vi "glueAlignPinInsert.vi"() -> ()   [LabVIEW 2015]
uses:
  GlobalPath.vi
  GlobalData.vi
  GlobalVi.vi
panel:
  in  "ptfe 41":bool caption="Manually push down the two pins of the vertical positioning tool to insert them in the holes of the plates"
  out "PanelName":string
  in  "ptfe 33":bool caption="Remove the electroerosion pin and the precision rod"
  in  "ptfe 10":bool caption="Place and screw the blocking plate to the vertical positioning tool to keep the pin orthogonality during the curing of the glue"
  in  "ptfe 40":bool caption="Insert the electroerosition pin in the slotted insert and the precision rod in the circular insert"
  in  "ptfe 38":bool caption="Check the planarity of the tool with the gauge machine"
  in  "ptfe 37":bool caption="Tighten the three screws to block the vertical positioning tool in place"
  in  "ptfe 35":bool caption="Position the vertical positioning tool on the reference plate against with its positioning pins"
  in  "ptfe 34":bool caption="Deposit the glue on the stainless steel slotted and circular insert groove"
  in  "ptfe 32":bool caption="Position the two inserts in the dedicated holes on the panel"
  in  "ptfe 26":bool caption="Position the panel on the table"
  in  "ptfe 25":bool caption="Move the panel away from the table"
  in  "ptfe 24":bool caption="Lift the panel from the table"
  in  "ptfe 23":bool caption="Switch on the vacuum on the machine"
  in  "ptfe 22":bool caption="Lower the machine on the panel"
  in  "ptfe 21":bool caption="Move the rotating machine on top of the panel"
  in  "Done ?":bool
  in  "ptfe 20":bool caption="Wait 24h for the glue to cure"
  in  "ptfe 19":bool caption="Position the reinforcing washers on the emerging part of the alignment inserts"
  in  "ptfe 18":bool caption="Deposit the glue on the emerging part of the alignment inserts using a thin needle"
  in  "ptfe 17":bool caption="Rotate the panel so that it's back side is up"
  in  "ptfe 16":bool caption="Switch off the vacuum"
  in  "ptfe 15":bool caption="Remove the three vertical positioning tools, blocking plates and positioning pins"
  in  "ptfe 14":bool caption="Wait 24h for the glue to cure"
  in  "ptfe 2":bool caption="Check that the vacuum is on"
  # "Gluing of Alignment Pin/Insert"
  # "ETA PANEL \nINSTRUCTIONS"
  # "GLUING OF THE SLOTTED BRASS AND CIRCULAR BRASS INSERT"
  # "Add info on enumeration"
  # "COMMON PROCEDURE"
  # "GLUE CURING OF THE TWO PINS AND INSERT"
  # "GLUING OF REINFORCING WASHERS ON PANEL BACK SIDE"
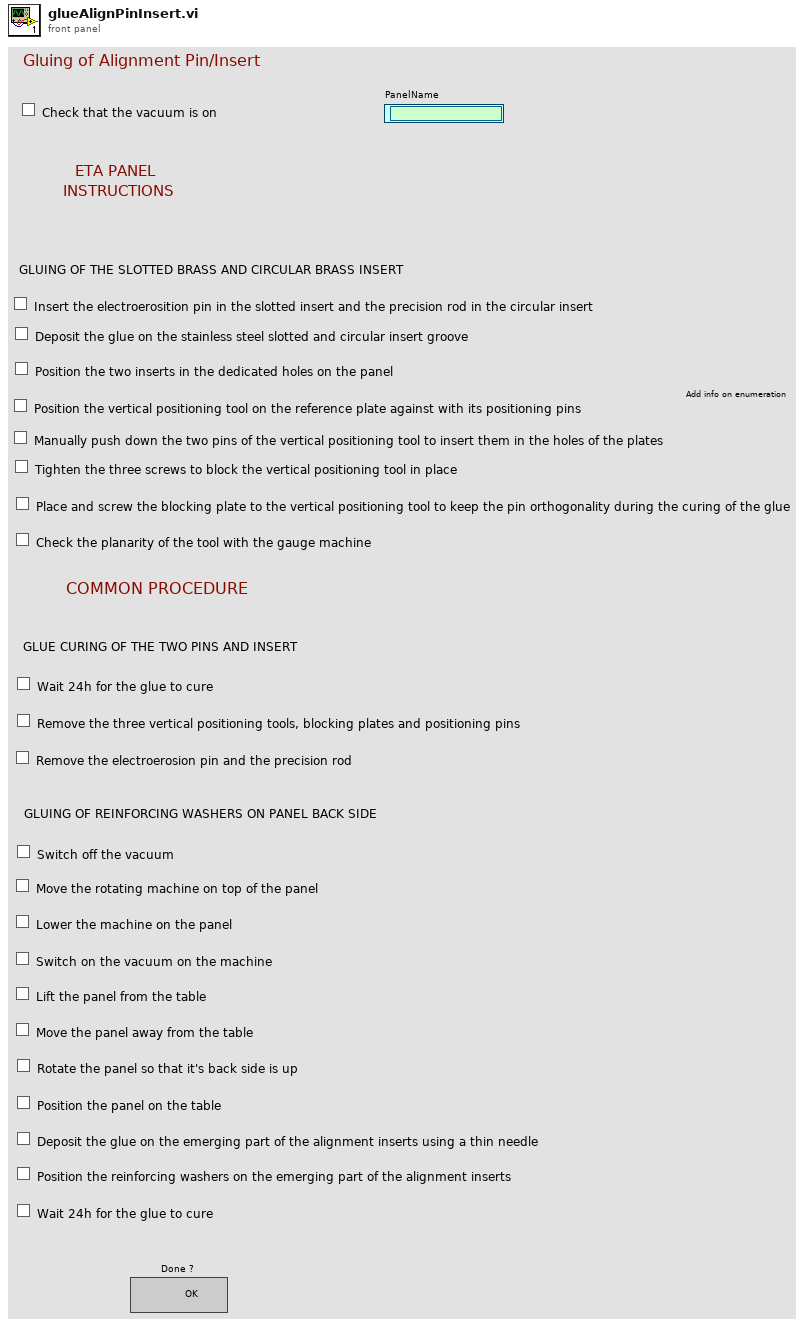
[diagram p1: front panel]
types:
  T1 = enum16{"open", "replace", "create", "open or create", "replace or create", "replace or create with confirmation"}
  T2 = enum32{"Bad", "Idle", "Run top level", "Running"}
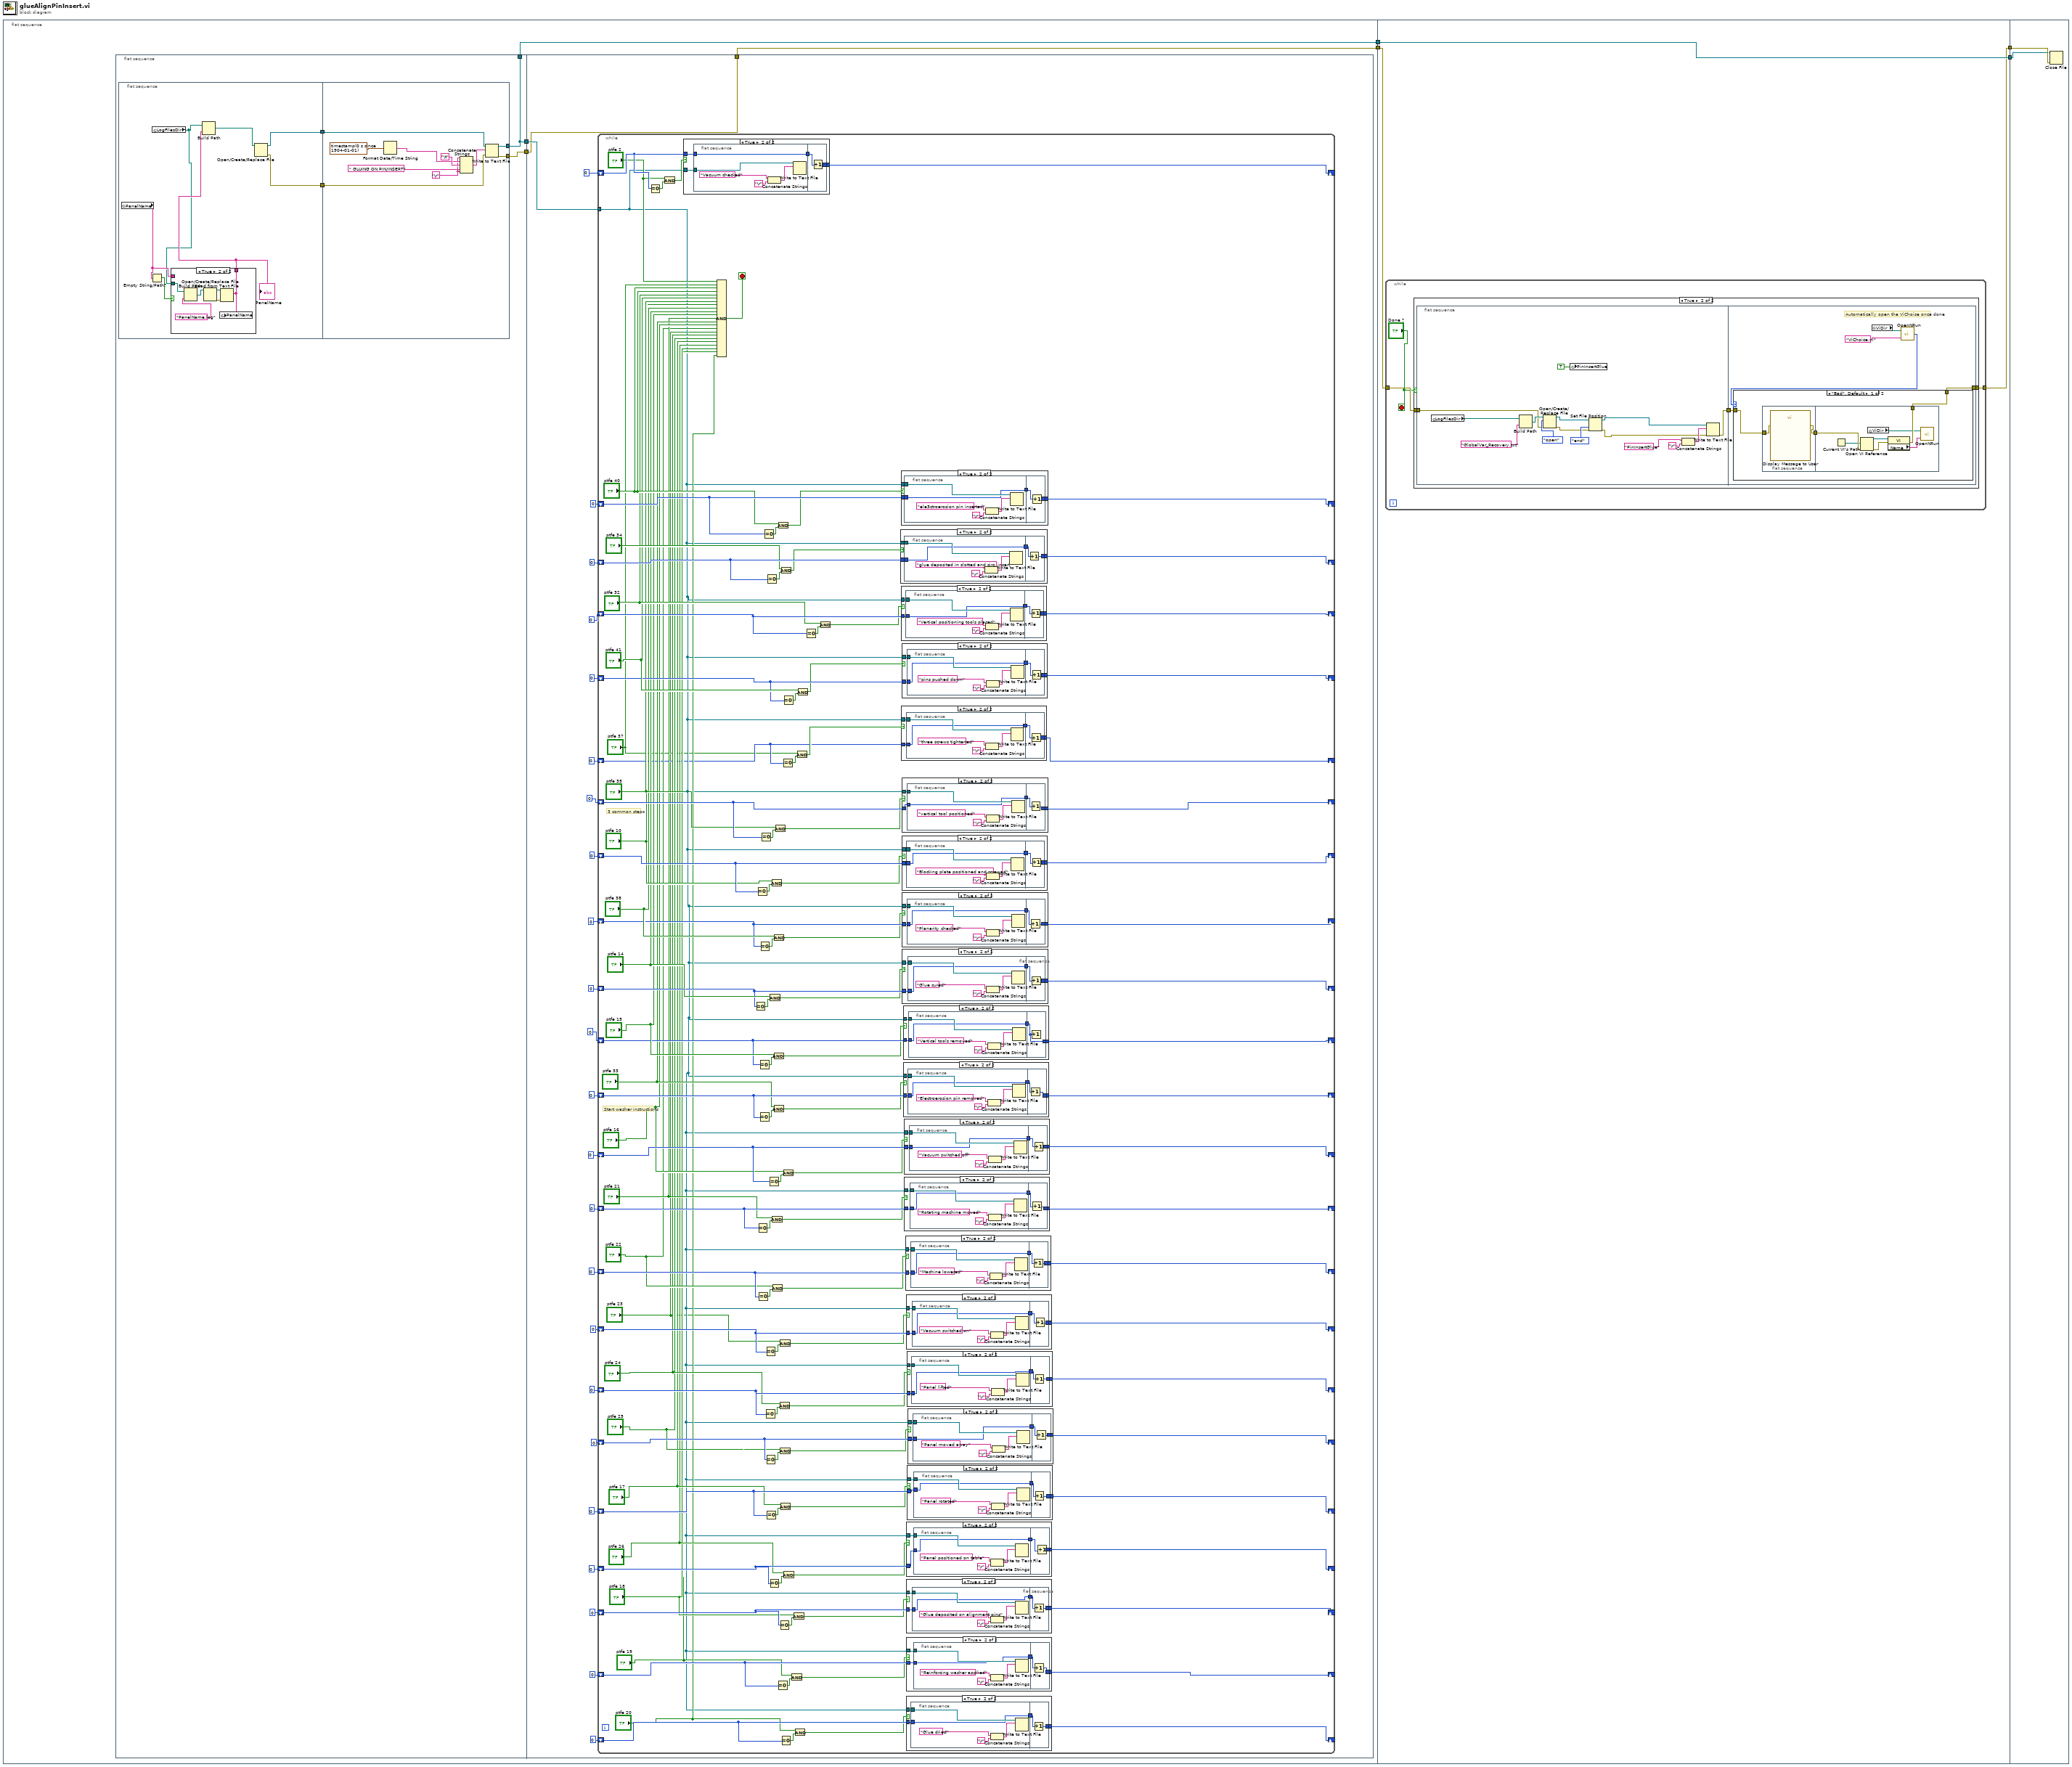
[diagram p0: block diagram]
diagram:
  n1 = flat-sequence {
    tunnel: [w5] -> w3
    tunnel: [w7] -> w2
    tunnel: [w454] -> w4
    tunnel: w3 -> [w455]
    tunnel: w2 -> [w456]
    tunnel: [w456] -> w1
    tunnel: w4 -> [w500]
    tunnel: w1 -> [w499]
    frame #0 {
      n2 = flat-sequence {
        tunnel: [w11] -> w8
        tunnel: [w11] -> w7
        tunnel: [w9] -> w6
        tunnel: w8 -> [w61]
        tunnel: w6 -> [w60]
        tunnel: [w60] -> w5
        frame #0 {
          n3 = flat-sequence {
            tunnel: [w18] -> w12
            tunnel: [w17] -> w10
            tunnel: w12 -> [w31]
            tunnel: [w30] -> w11
            tunnel: [w29] -> w9
            tunnel: w10 -> [w28]
            frame #0 {
              n4 = global read "GlobalData.vi" "PanelName"() -> (w16:string)
              n5 = Empty String/Path?(string/path=w16) -> (empty?=w15:bool)
              n6 = global read "GlobalPath.vi" "LogFilesDir"() -> (w13:path)
              n7 = case shown="True" w15 {
                tunnel: w13 -> [_ w26]
                tunnel: [w20 w21] -> w14
                tunnel: w16 -> [w20 _]
                frame False {
                }
                frame True {
                  n8 = Build Path(base path=w26, name or relative path="PanelName.log") -> (appended path=w25:path)
                  n9 = Open/Create/Replace File(file path (use dialog)=w25) -> (refnum out=w22:refnum<file>, error out=w23:errorcluster)  [unwired: 5 in, 1 out]
                  n10 = Read from Text File(file (use dialog)=w22, error in=w23) -> (text=w21:string)  [unwired: 2 in, 3 out]
                  n11 = global write "GlobalData.vi" "PanelName"(w21) -> ()
                }
              }
              "PanelName" <- w14
              n12 = Build Path(base path=w13, name or relative path=w14) -> (appended path=w19:path)
              n13 = Open/Create/Replace File(file path (use dialog)=w19) -> (refnum out=w18:refnum<file>, error out=w17:errorcluster)  [unwired: 5 in, 1 out]
            }
            frame #1 {
              w27 = "\r"
              n14 = Format Date/Time String(seconds (now)=timestamp(0 s since 1904-01-01)) -> (date/time string=w34:string)  [unwired: 2 in]
              n15 = Concatenate Strings(w27, w34, "\t", " GLUING ON PIN/INSERT", w27) -> (w32:string)
              n16 = Write to Text File(file (use dialog)=w31, text=w32, error in=w28) -> (refnum out=w30:refnum<file>, error out=w29:errorcluster)  [unwired: 1 in, 1 out]
            }
          }
        }
        frame #1 {
          n17 = while {
            tunnel: w61 -> [w67]
            shift-right: [w177] -> _
            shift-left: 0 -> [w154]
            shift-right: [w176] -> _
            shift-left: 0 -> [w146]
            shift-right: [w175] -> _
            shift-left: 0 -> [w145]
            shift-right: [w174] -> _
            shift-left: 0 -> [w144]
            shift-right: [w173] -> _
            shift-left: 0 -> [w136]
            shift-right: [w172] -> _
            shift-left: 0 -> [w134]
            shift-right: [w171] -> _
            shift-left: 0 -> [w126]
            shift-right: [w170] -> _
            shift-left: 0 -> [w122]
            shift-right: [w169] -> _
            shift-left: 0 -> [w119]
            shift-right: [w168] -> _
            shift-left: 0 -> [w116]
            shift-right: [w167] -> _
            shift-left: 0 -> [w114]
            shift-right: [w166] -> _
            shift-left: 0 -> [w103]
            shift-right: [w165] -> _
            shift-left: 0 -> [w102]
            shift-right: [w164] -> _
            shift-left: 0 -> [w101]
            shift-right: [w163] -> _
            shift-left: 0 -> [w100]
            shift-right: [w162] -> _
            shift-left: 0 -> [w99]
            shift-right: [w161] -> _
            shift-left: 0 -> [w98]
            shift-right: [w160] -> _
            shift-left: 0 -> [w97]
            shift-right: [w159] -> _
            shift-left: 0 -> [w96]
            shift-right: [w158] -> _
            shift-left: 0 -> [w95]
            shift-right: [w157] -> _
            shift-left: 0 -> [w75]
            shift-right: [w156] -> _
            shift-left: 0 -> [w74]
            shift-right: [w65] -> _
            shift-left: 0 -> [w66]
            stop <- w178 stop-if-true
            # "3 common steps"
            # "Start washer instructions"
            n18 = Equal To 0?(x=w154) -> (x = 0?=w155:bool)
            n19 = And(x="ptfe 2", y=w155) -> (x .and. y?=w152:bool)
            n20 = case shown="True" w152 {
              tunnel: w67 -> [_ w446]
              tunnel: w154 -> [w442 w445]
              tunnel: [w442 w443] -> w177
              frame False {
              }
              frame True {
                n21 = flat-sequence {
                  tunnel: w446 -> [w448]
                  tunnel: w445 -> [w447]
                  tunnel: [w447] -> w444
                  tunnel: w444 -> [w453]
                  tunnel: [w452] -> w443
                  frame #0 {
                    n22 = Concatenate Strings("Vacuum checked", "\r") -> (w451:string)
                    n23 = Write to Text File(file (use dialog)=w448, text=w451) -> ()  [unwired: 2 in, 3 out]
                  }
                  frame #1 {
                    n24 = Increment(x=w453) -> (x+1=w452:i32)
                  }
                }
              }
            }
            n25 = Compound Arithmetic op=AND("ptfe 2", "ptfe 37", "ptfe 40", "ptfe 40", "ptfe 32", "ptfe 41", "ptfe 35", "ptfe 10", "ptfe 38", "ptfe 14", "ptfe 15", "ptfe 21", "ptfe 33", "ptfe 16", "ptfe 22", "ptfe 23", "ptfe 24", "ptfe 25", "ptfe 17", "ptfe 26", "ptfe 18", "ptfe 19", "ptfe 20") -> (w178:bool)
            n26 = Equal To 0?(x=w119) -> (x = 0?=w129:bool)
            n27 = Equal To 0?(x=w126) -> (x = 0?=w131:bool)
            n28 = Equal To 0?(x=w102) -> (x = 0?=w111:bool)
            n29 = Equal To 0?(x=w101) -> (x = 0?=w110:bool)
            n30 = Equal To 0?(x=w116) -> (x = 0?=w128:bool)
            n31 = Equal To 0?(x=w114) -> (x = 0?=w127:bool)
            n32 = Equal To 0?(x=w122) -> (x = 0?=w130:bool)
            n33 = Equal To 0?(x=w134) -> (x = 0?=w147:bool)
            n34 = Equal To 0?(x=w146) -> (x = 0?=w151:bool)
            n35 = Equal To 0?(x=w99) -> (x = 0?=w108:bool)
            n36 = Equal To 0?(x=w100) -> (x = 0?=w109:bool)
            n37 = Equal To 0?(x=w98) -> (x = 0?=w107:bool)
            n38 = Equal To 0?(x=w97) -> (x = 0?=w106:bool)
            n39 = Equal To 0?(x=w145) -> (x = 0?=w150:bool)
            n40 = Equal To 0?(x=w103) -> (x = 0?=w112:bool)
            n41 = Equal To 0?(x=w96) -> (x = 0?=w105:bool)
            n42 = And(x="ptfe 14", y=w129) -> (x .and. y?=w118:bool)
            n43 = And(x="ptfe 10", y=w131) -> (x .and. y?=w124:bool)
            n44 = And(x="ptfe 21", y=w111) -> (x .and. y?=w90:bool)
            n45 = And(x="ptfe 22", y=w110) -> (x .and. y?=w88:bool)
            n46 = And(x="ptfe 15", y=w128) -> (x .and. y?=w115:bool)
            n47 = And(x="ptfe 33", y=w127) -> (x .and. y?=w113:bool)
            n48 = And(x="ptfe 38", y=w130) -> (x .and. y?=w121:bool)
            n49 = And(x="ptfe 35", y=w147) -> (x .and. y?=w132:bool)
            n50 = Equal To 0?(x=w75) -> (x = 0?=w77:bool)
            n51 = And(x="ptfe 40", y=w151) -> (x .and. y?=w142:bool)
            n52 = And(x="ptfe 24", y=w108) -> (x .and. y?=w86:bool)
            n53 = Equal To 0?(x=w95) -> (x = 0?=w104:bool)
            n54 = And(x="ptfe 23", y=w109) -> (x .and. y?=w62:bool)
            n55 = And(x="ptfe 25", y=w107) -> (x .and. y?=w84:bool)
            n56 = And(x="ptfe 17", y=w106) -> (x .and. y?=w82:bool)
            n57 = Equal To 0?(x=w74) -> (x = 0?=w76:bool)
            n58 = And(x="ptfe 34", y=w150) -> (x .and. y?=w140:bool)
            n59 = Equal To 0?(x=w66) -> (x = 0?=w69:bool)
            n60 = Equal To 0?(x=w136) -> (x = 0?=w148:bool)
            n61 = And(x="ptfe 16", y=w112) -> (x .and. y?=w92:bool)
            n62 = And(x="ptfe 26", y=w105) -> (x .and. y?=w80:bool)
            n63 = And(x="ptfe 19", y=w77) -> (x .and. y?=w73:bool)
            n64 = And(x="ptfe 18", y=w104) -> (x .and. y?=w78:bool)
            n65 = And(x="ptfe 20", y=w76) -> (x .and. y?=w72:bool)
            n66 = And(x="ptfe 37", y=w69) -> (x .and. y?=w68:bool)
            n67 = And(x="ptfe 41", y=w148) -> (x .and. y?=w135:bool)
            n68 = Equal To 0?(x=w144) -> (x = 0?=w149:bool)
            n69 = And(x="ptfe 32", y=w149) -> (x .and. y?=w139:bool)
            n70 = case shown="True" w140 {
              tunnel: w67 -> [_ w422]
              tunnel: w145 -> [w418 w420]
              tunnel: [w418 w419] -> w175
              frame False {
              }
              frame True {
                n71 = flat-sequence {
                  tunnel: w422 -> [w424]
                  tunnel: [w423] -> w421
                  tunnel: w420 -> [w423]
                  tunnel: w421 -> [w429]
                  tunnel: [w428] -> w419
                  frame #0 {
                    n72 = Concatenate Strings("glue deposited in slotted and circ. insert", "\r") -> (w427:string)
                    n73 = Write to Text File(file (use dialog)=w424, text=w427) -> ()  [unwired: 2 in, 3 out]
                  }
                  frame #1 {
                    n74 = Increment(x=w429) -> (x+1=w428:i32)
                  }
                }
              }
            }
            n75 = case shown="True" w142 {
              tunnel: w67 -> [_ w434]
              tunnel: w146 -> [w430 w433]
              tunnel: [w430 w431] -> w176
              frame False {
              }
              frame True {
                n76 = flat-sequence {
                  tunnel: w434 -> [w436]
                  tunnel: w433 -> [w435]
                  tunnel: [w435] -> w432
                  tunnel: w432 -> [w441]
                  tunnel: [w440] -> w431
                  frame #0 {
                    n77 = Concatenate Strings("ele3ctroerosion pin inserted", "\r") -> (w439:string)
                    n78 = Write to Text File(file (use dialog)=w436, text=w439) -> ()  [unwired: 2 in, 3 out]
                  }
                  frame #1 {
                    n79 = Increment(x=w441) -> (x+1=w440:i32)
                  }
                }
              }
            }
            n80 = case shown="True" w139 {
              tunnel: w67 -> [_ w410]
              tunnel: w144 -> [w406 w408]
              tunnel: [w406 w407] -> w174
              frame False {
              }
              frame True {
                n81 = flat-sequence {
                  tunnel: w410 -> [w412]
                  tunnel: [w411] -> w409
                  tunnel: w408 -> [w411]
                  tunnel: w409 -> [w417]
                  tunnel: [w416] -> w407
                  frame #0 {
                    n82 = Concatenate Strings("Vertical positioning tools placed", "\r") -> (w415:string)
                    n83 = Write to Text File(file (use dialog)=w412, text=w415) -> ()  [unwired: 2 in, 3 out]
                  }
                  frame #1 {
                    n84 = Increment(x=w417) -> (x+1=w416:i32)
                  }
                }
              }
            }
            n85 = case shown="True" w68 {
              tunnel: w67 -> [_ w183]
              tunnel: w66 -> [w179 w181]
              tunnel: [w179 w180] -> w65
              frame False {
              }
              frame True {
                n86 = flat-sequence {
                  tunnel: w183 -> [w185]
                  tunnel: [w184] -> w182
                  tunnel: w181 -> [w184]
                  tunnel: w182 -> [w190]
                  tunnel: [w189] -> w180
                  frame #0 {
                    n87 = Concatenate Strings("three screws tightened", "\r") -> (w188:string)
                    n88 = Write to Text File(file (use dialog)=w185, text=w188) -> ()  [unwired: 2 in, 3 out]
                  }
                  frame #1 {
                    n89 = Increment(x=w190) -> (x+1=w189:i32)
                  }
                }
              }
            }
            n90 = case shown="True" w135 {
              tunnel: w67 -> [_ w362]
              tunnel: w136 -> [w358 w360]
              tunnel: [w358 w359] -> w173
              frame False {
              }
              frame True {
                n91 = flat-sequence {
                  tunnel: w362 -> [w364]
                  tunnel: [w363] -> w361
                  tunnel: w360 -> [w363]
                  tunnel: w361 -> [w369]
                  tunnel: [w368] -> w359
                  frame #0 {
                    n92 = Concatenate Strings("pins pushed down", "\r") -> (w367:string)
                    n93 = Write to Text File(file (use dialog)=w364, text=w367) -> ()  [unwired: 2 in, 3 out]
                  }
                  frame #1 {
                    n94 = Increment(x=w369) -> (x+1=w368:i32)
                  }
                }
              }
            }
            n95 = case shown="True" w124 {
              tunnel: w67 -> [_ w386]
              tunnel: w126 -> [w382 w385]
              tunnel: [w382 w383] -> w171
              frame False {
              }
              frame True {
                n96 = flat-sequence {
                  tunnel: w386 -> [w388]
                  tunnel: w385 -> [w387]
                  tunnel: [w387] -> w384
                  tunnel: w384 -> [w393]
                  tunnel: [w392] -> w383
                  frame #0 {
                    n97 = Concatenate Strings("Blocking plate positioned and screwed", "\r") -> (w391:string)
                    n98 = Write to Text File(file (use dialog)=w388, text=w391) -> ()  [unwired: 2 in, 3 out]
                  }
                  frame #1 {
                    n99 = Increment(x=w393) -> (x+1=w392:i32)
                  }
                }
              }
            }
            n100 = case shown="True" w132 {
              tunnel: w67 -> [_ w398]
              tunnel: w134 -> [w394 w397]
              tunnel: [w394 w395] -> w172
              frame False {
              }
              frame True {
                n101 = flat-sequence {
                  tunnel: w398 -> [w400]
                  tunnel: w397 -> [w399]
                  tunnel: [w399] -> w396
                  tunnel: w396 -> [w405]
                  tunnel: [w404] -> w395
                  frame #0 {
                    n102 = Concatenate Strings("vertical tool positioned", "\r") -> (w403:string)
                    n103 = Write to Text File(file (use dialog)=w400, text=w403) -> ()  [unwired: 2 in, 3 out]
                  }
                  frame #1 {
                    n104 = Increment(x=w405) -> (x+1=w404:i32)
                  }
                }
              }
            }
            n105 = case shown="True" w121 {
              tunnel: w67 -> [_ w374]
              tunnel: w122 -> [w370 w372]
              tunnel: [w370 w371] -> w170
              frame False {
              }
              frame True {
                n106 = flat-sequence {
                  tunnel: w374 -> [w376]
                  tunnel: [w375] -> w373
                  tunnel: w372 -> [w375]
                  tunnel: w373 -> [w381]
                  tunnel: [w380] -> w371
                  frame #0 {
                    n107 = Concatenate Strings("Planarity checked", "\r") -> (w379:string)
                    n108 = Write to Text File(file (use dialog)=w376, text=w379) -> ()  [unwired: 2 in, 3 out]
                  }
                  frame #1 {
                    n109 = Increment(x=w381) -> (x+1=w380:i32)
                  }
                }
              }
            }
            n110 = case shown="True" w118 {
              tunnel: w67 -> [_ w350]
              tunnel: w119 -> [w346 w348]
              tunnel: [w346 w347] -> w169
              frame False {
              }
              frame True {
                n111 = flat-sequence {
                  tunnel: w350 -> [w352]
                  tunnel: [w351] -> w349
                  tunnel: w348 -> [w351]
                  tunnel: w349 -> [w357]
                  tunnel: [w356] -> w347
                  frame #0 {
                    n112 = Concatenate Strings("Glue cured", "\r") -> (w355:string)
                    n113 = Write to Text File(file (use dialog)=w352, text=w355) -> ()  [unwired: 2 in, 3 out]
                  }
                  frame #1 {
                    n114 = Increment(x=w357) -> (x+1=w356:i32)
                  }
                }
              }
            }
            n115 = case shown="True" w115 {
              tunnel: w67 -> [_ w339]
              tunnel: w116 -> [w335 w337]
              tunnel: [w335 w336] -> w168
              frame False {
              }
              frame True {
                n116 = flat-sequence {
                  tunnel: w339 -> [w341]
                  tunnel: [w340] -> w338
                  tunnel: w337 -> [w340]
                  tunnel: w338 -> [w345]
                  tunnel: [w345] -> w336
                  frame #0 {
                    n117 = Concatenate Strings("Vertical tools removed", "\r") -> (w344:string)
                    n118 = Write to Text File(file (use dialog)=w341, text=w344) -> ()  [unwired: 2 in, 3 out]
                  }
                  frame #1 {
                    n119 = Increment(x=w345) -> ()  [unwired: 1 out]
                  }
                }
              }
            }
            n120 = case shown="True" w113 {
              tunnel: w67 -> [_ w327]
              tunnel: w114 -> [w323 w325]
              tunnel: [w323 w324] -> w167
              frame False {
              }
              frame True {
                n121 = flat-sequence {
                  tunnel: w327 -> [w329]
                  tunnel: [w328] -> w326
                  tunnel: w325 -> [w328]
                  tunnel: w326 -> [w334]
                  tunnel: [w333] -> w324
                  frame #0 {
                    n122 = Concatenate Strings("Electroerosion pin removed", "\r") -> (w332:string)
                    n123 = Write to Text File(file (use dialog)=w329, text=w332) -> ()  [unwired: 2 in, 3 out]
                  }
                  frame #1 {
                    n124 = Increment(x=w334) -> (x+1=w333:i32)
                  }
                }
              }
            }
            n125 = case shown="True" w92 {
              tunnel: w67 -> [_ w315]
              tunnel: w103 -> [w311 w313]
              tunnel: [w311 w312] -> w166
              frame False {
              }
              frame True {
                n126 = flat-sequence {
                  tunnel: w315 -> [w317]
                  tunnel: [w316] -> w314
                  tunnel: w313 -> [w316]
                  tunnel: w314 -> [w322]
                  tunnel: [w321] -> w312
                  frame #0 {
                    n127 = Concatenate Strings("Vacuum switched off", "\r") -> (w320:string)
                    n128 = Write to Text File(file (use dialog)=w317, text=w320) -> ()  [unwired: 2 in, 3 out]
                  }
                  frame #1 {
                    n129 = Increment(x=w322) -> (x+1=w321:i32)
                  }
                }
              }
            }
            n130 = case shown="True" w90 {
              tunnel: w67 -> [_ w303]
              tunnel: w102 -> [w299 w301]
              tunnel: [w299 w300] -> w165
              frame False {
              }
              frame True {
                n131 = flat-sequence {
                  tunnel: w303 -> [w305]
                  tunnel: [w304] -> w302
                  tunnel: w301 -> [w304]
                  tunnel: w302 -> [w310]
                  tunnel: [w309] -> w300
                  frame #0 {
                    n132 = Concatenate Strings("Rotating machine moved", "\r") -> (w308:string)
                    n133 = Write to Text File(file (use dialog)=w305, text=w308) -> ()  [unwired: 2 in, 3 out]
                  }
                  frame #1 {
                    n134 = Increment(x=w310) -> (x+1=w309:i32)
                  }
                }
              }
            }
            n135 = case shown="True" w88 {
              tunnel: w67 -> [_ w291]
              tunnel: w101 -> [w287 w289]
              tunnel: [w287 w288] -> w164
              frame False {
              }
              frame True {
                n136 = flat-sequence {
                  tunnel: w291 -> [w293]
                  tunnel: [w292] -> w290
                  tunnel: w289 -> [w292]
                  tunnel: w290 -> [w298]
                  tunnel: [w297] -> w288
                  frame #0 {
                    n137 = Concatenate Strings("Machine lowered", "\r") -> (w296:string)
                    n138 = Write to Text File(file (use dialog)=w293, text=w296) -> ()  [unwired: 2 in, 3 out]
                  }
                  frame #1 {
                    n139 = Increment(x=w298) -> (x+1=w297:i32)
                  }
                }
              }
            }
            n140 = case shown="True" w62 {
              tunnel: w67 -> [_ w279]
              tunnel: w100 -> [w275 w277]
              tunnel: [w275 w276] -> w163
              frame False {
              }
              frame True {
                n141 = flat-sequence {
                  tunnel: w279 -> [w281]
                  tunnel: [w280] -> w278
                  tunnel: w277 -> [w280]
                  tunnel: w278 -> [w286]
                  tunnel: [w285] -> w276
                  frame #0 {
                    n142 = Concatenate Strings("Vacuum switched on", "\r") -> (w284:string)
                    n143 = Write to Text File(file (use dialog)=w281, text=w284) -> ()  [unwired: 2 in, 3 out]
                  }
                  frame #1 {
                    n144 = Increment(x=w286) -> (x+1=w285:i32)
                  }
                }
              }
            }
            n145 = case shown="True" w78 {
              tunnel: w67 -> [_ w231]
              tunnel: w95 -> [w227 w229]
              tunnel: [w227 w228] -> w158
              frame False {
              }
              frame True {
                n146 = flat-sequence {
                  tunnel: w231 -> [w233]
                  tunnel: [w232] -> w230
                  tunnel: w229 -> [w232]
                  tunnel: w230 -> [w238]
                  tunnel: [w237] -> w228
                  frame #0 {
                    n147 = Concatenate Strings("Glue deposited on alignment pins", "\r") -> (w236:string)
                    n148 = Write to Text File(file (use dialog)=w233, text=w236) -> ()  [unwired: 2 in, 3 out]
                  }
                  frame #1 {
                    n149 = Increment(x=w238) -> (x+1=w237:i32)
                  }
                }
              }
            }
            n150 = case shown="True" w72 {
              tunnel: w67 -> [_ w207]
              tunnel: w74 -> [w203 w206]
              tunnel: [w203 w204] -> w156
              frame False {
              }
              frame True {
                n151 = flat-sequence {
                  tunnel: w207 -> [w209]
                  tunnel: w206 -> [w208]
                  tunnel: [w208] -> w205
                  tunnel: w205 -> [w214]
                  tunnel: [w213] -> w204
                  frame #0 {
                    n152 = Concatenate Strings("Glue dried", "\r") -> (w212:string)
                    n153 = Write to Text File(file (use dialog)=w209, text=w212) -> ()  [unwired: 2 in, 3 out]
                  }
                  frame #1 {
                    n154 = Increment(x=w214) -> (x+1=w213:i32)
                  }
                }
              }
            }
            n155 = case shown="True" w80 {
              tunnel: w67 -> [_ w243]
              tunnel: w96 -> [w239 w242]
              tunnel: [w239 w240] -> w159
              frame False {
              }
              frame True {
                n156 = flat-sequence {
                  tunnel: w243 -> [w245]
                  tunnel: w242 -> [w244]
                  tunnel: [w244] -> w241
                  tunnel: w241 -> [w250]
                  tunnel: [w249] -> w240
                  frame #0 {
                    n157 = Concatenate Strings("Panel positioned on table", "\r") -> (w248:string)
                    n158 = Write to Text File(file (use dialog)=w245, text=w248) -> ()  [unwired: 2 in, 3 out]
                  }
                  frame #1 {
                    n159 = Increment(x=w250) -> (x+1=w249:i32)
                  }
                }
              }
            }
            n160 = case shown="True" w73 {
              tunnel: w67 -> [_ w219]
              tunnel: w75 -> [w215 w217]
              tunnel: [w215 w216] -> w157
              frame False {
              }
              frame True {
                n161 = flat-sequence {
                  tunnel: w219 -> [w221]
                  tunnel: [w220] -> w218
                  tunnel: w217 -> [w220]
                  tunnel: w218 -> [w226]
                  tunnel: [w225] -> w216
                  frame #0 {
                    n162 = Concatenate Strings("Reinforcing washer applied", "\r") -> (w224:string)
                    n163 = Write to Text File(file (use dialog)=w221, text=w224) -> ()  [unwired: 2 in, 3 out]
                  }
                  frame #1 {
                    n164 = Increment(x=w226) -> (x+1=w225:i32)
                  }
                }
              }
            }
            n165 = case shown="True" w86 {
              tunnel: w67 -> [_ w267]
              tunnel: w99 -> [w263 w265]
              tunnel: [w263 w264] -> w162
              frame False {
              }
              frame True {
                n166 = flat-sequence {
                  tunnel: w267 -> [w269]
                  tunnel: [w268] -> w266
                  tunnel: w265 -> [w268]
                  tunnel: w266 -> [w274]
                  tunnel: [w273] -> w264
                  frame #0 {
                    n167 = Concatenate Strings("Panel lifted", "\r") -> (w272:string)
                    n168 = Write to Text File(file (use dialog)=w269, text=w272) -> ()  [unwired: 2 in, 3 out]
                  }
                  frame #1 {
                    n169 = Increment(x=w274) -> (x+1=w273:i32)
                  }
                }
              }
            }
            n170 = case shown="True" w82 {
              tunnel: w67 -> [_ w195]
              tunnel: w97 -> [w191 w194]
              tunnel: [w191 w192] -> w160
              frame False {
              }
              frame True {
                n171 = flat-sequence {
                  tunnel: w195 -> [w197]
                  tunnel: w194 -> [w196]
                  tunnel: [w196] -> w193
                  tunnel: w193 -> [w202]
                  tunnel: [w201] -> w192
                  frame #0 {
                    n172 = Concatenate Strings("Panel rotated", "\r") -> (w200:string)
                    n173 = Write to Text File(file (use dialog)=w197, text=w200) -> ()  [unwired: 2 in, 3 out]
                  }
                  frame #1 {
                    n174 = Increment(x=w202) -> (x+1=w201:i32)
                  }
                }
              }
            }
            n175 = case shown="True" w84 {
              tunnel: w67 -> [_ w255]
              tunnel: w98 -> [w251 w253]
              tunnel: [w251 w252] -> w161
              frame False {
              }
              frame True {
                n176 = flat-sequence {
                  tunnel: w255 -> [w257]
                  tunnel: [w256] -> w254
                  tunnel: w253 -> [w256]
                  tunnel: w254 -> [w262]
                  tunnel: [w261] -> w252
                  frame #0 {
                    n177 = Concatenate Strings("Panel moved away", "\r") -> (w260:string)
                    n178 = Write to Text File(file (use dialog)=w257, text=w260) -> ()  [unwired: 2 in, 3 out]
                  }
                  frame #1 {
                    n179 = Increment(x=w262) -> (x+1=w261:i32)
                  }
                }
              }
            }
          }
        }
      }
    }
    frame #1 {
      n180 = while {
        tunnel: [w459] -> w454
        tunnel: w455 -> [w458]
        stop <- "Done ?" stop-if-true
        n181 = case shown="True" "Done ?" {
          tunnel: [w460 w463] -> w459
          tunnel: w458 -> [w460 w462]
          frame False {
          }
          frame True {
            n182 = flat-sequence {
              tunnel: w462 -> [w467]
              tunnel: [w466] -> w461
              tunnel: [w480] -> w463
              tunnel: w461 -> [w479]
              frame #0 {
                n183 = global read "GlobalPath.vi" "LogFilesDir"() -> (w464:path)
                n184 = Build Path(base path=w464, name or relative path="GlobalVar_Recovery.txt") -> (appended path=w476:path)
                n185 = Open/Create/Replace File(file path (use dialog)=w476, error in=w467, operation (0:open)=T1."open") -> (refnum out=w472:refnum<file>, error out=w473:errorcluster)  [unwired: 3 in, 1 out]
                n186 = global write "GlobalVi.vi" "PinInsertGlue"(TRUE) -> ()
                n187 = Set File Position(refnum=w472, from (0:start)=enum16{"start", "end", "current"}."end", error in=w473) -> (refnum out=w469:refnum<file>, error out=w468:errorcluster)  [unwired: 1 in]
                n188 = Concatenate Strings("PinInsertGlue", "\r") -> (w471:string)
                n189 = Write to Text File(file (use dialog)=w469, text=w471, error in=w468) -> (error out=w466:errorcluster)  [unwired: 1 in, 2 out]
              }
              frame #1 {
                # "Automatically open the ViChoise once done"
                n190 = global read "GlobalPath.vi" "ViDir"() -> (w483:path)
                n191 = call "OpenNRun.vi"("VI name"="ViChoice.vi", "ViDirPath"=w483) -> ("Execution:State"=w482:T2)
                n192 = case shown="\"Bad\", Default" w482 {
                  tunnel: [w484 w496] -> w480
                  tunnel: w479 -> [w485 w496]
                  frame "Bad", Default {
                    n193 = flat-sequence {
                      tunnel: w485 -> [w488]
                      tunnel: [w487] -> w486
                      tunnel: [w492] -> w484
                      tunnel: w486 -> [w491]
                      frame #0 {
                        n194 = call "Display Message to User"("error in (no error)"=w488) -> ("error out"=w487:errorcluster)  [unwired: 9 in, 1 out]
                      }
                      frame #1 {
                        n195 = Current VI's Path() -> (path=w489:path)
                        n196 = Open VI Reference(vi path=w489, error in (no error)=w491) -> (vi reference=w495:refnum<vi>, error out=w494:errorcluster)  [unwired: 4 in]
                        n197 = global read "GlobalPath.vi" "ViDir"() -> (w490:path)
                        n198 = property class="VI"(reference=w495, error in=w494) -> (error out=w492:errorcluster, "Name"=w493:string)  [unwired: 1 out]
                        n199 = call "OpenNRun.vi"("VI name"=w493, "ViDirPath"=w490) -> ()  [unwired: 1 out]
                      }
                    }
                  }
                  frame "Idle" {
                    n200 = Current VI's Path() -> (path=w497:path)
                    n201 = Strip Path(path=w497) -> (name=w498:string)  [unwired: 1 out]
                    n202 = call <vilib>:"Close Panel.vi"("VI name"=w498) -> ()  [unwired: 10 in, 1 out]
                  }
                }
              }
            }
          }
        }
      }
    }
    frame #2 {
      n203 = Close File(refnum=w499, error in=w500) -> ()  [unwired: 2 out]
    }
  }
